vi "Enable Output.vi"(7 "Enable Output (T: Enable)":bool=TRUE, 8 "error in (no error)":errorcluster, 11 "VISA resource name":refnum<visa-resource-name>) -> (0 "error out":errorcluster, 3 "VISA resource name out":refnum<visa-resource-name>)   [LabVIEW 2020, in "Template - Function Generator.lvlib"]
doc: "Enables or disables the output connector."
uses:
  <instrlib>/_Template - Function Generator/Template - Function Generator.lvlib
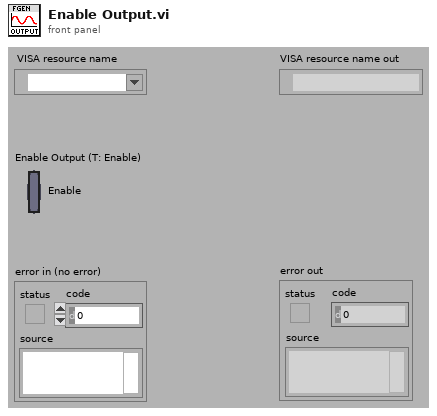
[diagram p1: front panel]
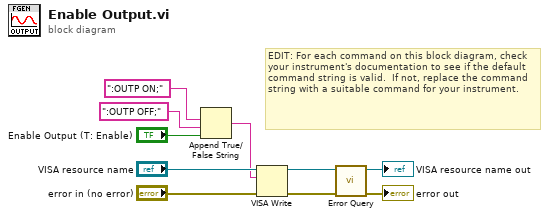
[diagram p0: block diagram]
diagram:
  # "EDIT: For each command on this block diagram, check your instrument's documentation to see if the default command string is valid.  If not, replace the command string with a suitable command for your instrument."
  n1 = Append True/False String(1:"Enable Output (T: Enable)", 2:":OUTP OFF;" ("true string"), 3:":OUTP ON;" ("true string")) -> (0:w5:string)  [unwired: 1 in]
  n2 = VISA Write(VISA resource name="VISA resource name", write buffer=w5, error in (no error)="error in (no error)") -> (VISA resource name out=w3:refnum<visa-resource-name>, error out=w4:errorcluster)  [unwired: 1 out]
  n3 = call <instrlib>:"Error Query.vi"("error in (no error)"=w4, "VISA resource name"=w3) -> ("error out"=→"error out":errorcluster, "VISA resource name out"=→"VISA resource name out":refnum<visa-resource-name>)  [unwired: 6 in, 2 out]
